vi "RG Configure Delay TDS3012C.vi"(8 "error in (no error)":errorcluster, 9 "Horizontal Delay (0 s)":dbl, 10 "Enable Delay (T: Enable)":bool=TRUE, 11 "VISA resource name":refnum<visa-resource-name>) -> (0 "error out":errorcluster, 3 "VISA resource name out":refnum<visa-resource-name>)   [LabVIEW 2017, in "Scope.lvlib" / "Tektronix DPO MSO 2000 4000 Series.lvlib"]
doc: "Configures the horizontal delay settings."
uses:
  Tektronix DPO MSO 2000 4000 Series.lvlib
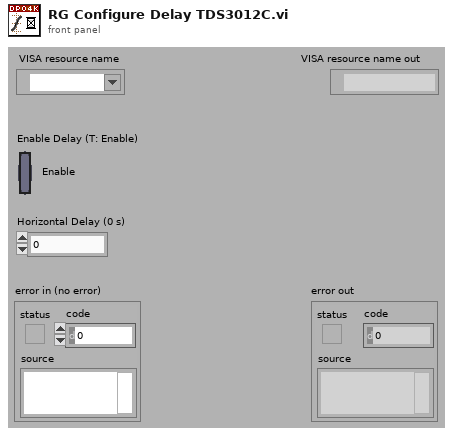
[diagram p1: front panel]
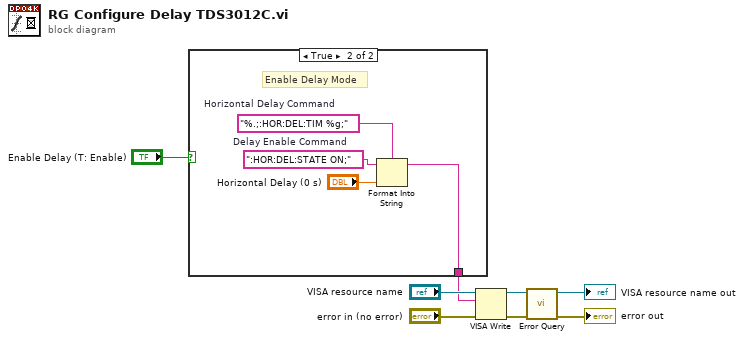
[diagram p0: block diagram]
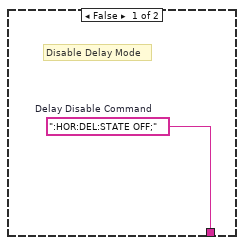
[diagram p2: hidden frame]
diagram:
  n1 = case shown="True" "Enable Delay (T: Enable)" {
    tunnel: [w9 w10] -> w1
    frame False {
      w9 = ":HOR:DEL:STATE OFF;"  # Delay Disable Command
      # "Disable Delay Mode"
    }
    frame True {
      w12 = ":HOR:DEL:STATE ON;"  # Delay Enable Command
      w13 = "%.;:HOR:DEL:TIM %g;"  # Horizontal Delay Command
      # "Enable Delay Mode"
      n2 = Format Into String(format string=w13, initial string=w12, "Horizontal Delay (0 s)") -> (resulting string=w10:string)  [unwired: 1 in, 1 out]
    }
  }
  n3 = VISA Write(VISA resource name="VISA resource name", write buffer=w1, error in (no error)="error in (no error)") -> (VISA resource name out=w4:refnum<visa-resource-name>, error out=w3:errorcluster)  [unwired: 1 out]
  n4 = call "Error Query.vi"("error in (no error)"=w3, "VISA resource name"=w4) -> ("error out"=→"error out":errorcluster, "VISA resource name out"=→"VISA resource name out":refnum<visa-resource-name>)  [unwired: 6 in, 2 out]
